vi "get remaining time budget.vi"(8 "error in":errorcluster, 10 "dt":u32=1, 11 "timing source in":refnum<class "ms timing source.lvclass">) -> (0 "error out":errorcluster, 2 "budget (ns)":u64, 3 "timing source out":refnum<class "ms timing source.lvclass">)   [LabVIEW 2013, in "ms timing source.lvclass"]
uses:
  ms timing source.lvclass
  ms timing source.lvclass/ms timing source.ctl
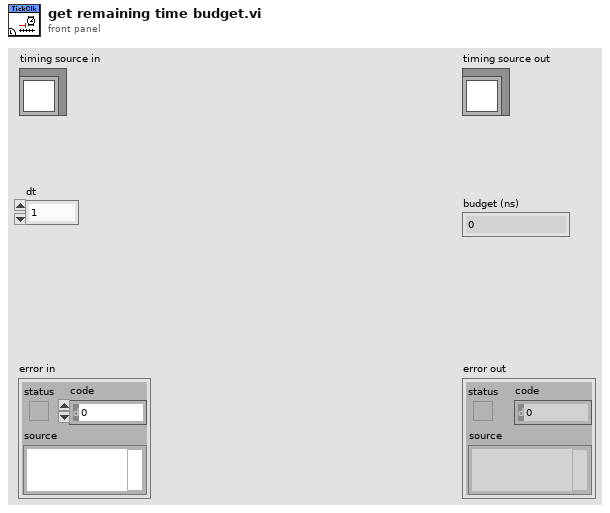
[diagram p1: front panel]
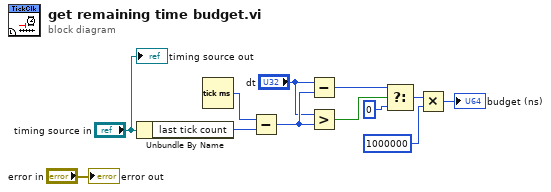
[diagram p0: block diagram]
diagram:
  n1 = Unbundle By Name("timing source in") -> ("last tick count"=w11:u32)
  n2 = Tick Count (ms)() -> (millisecond timer value=w1:u32)
  n3 = Subtract(x=w1, y=w11) -> (x-y=w9:u32)
  n4 = Subtract(x="dt", y=w9) -> (x-y=w8:u32)
  n5 = Greater?(x="dt", y=w9) -> (0:w10:bool)
  n6 = Select(t=w8, s=w10, f=u32 0) -> (s? t:f=w6:u32)
  n7 = Multiply(x=w6, y=u32 1000000) -> (x*y=→"budget (ns)":u32)
  "error out" <- "error in"
  "timing source out" <- "timing source in"
